vi "Add x.vi"(10 "x":sgl, 11 "Vector 2D in":refnum<class "Vector 2D.lvclass">) -> (3 "Vector 2D out":refnum<class "Vector 2D.lvclass">)   [LabVIEW 2021, in "Vector 2D.lvclass"]
uses:
  Vector 2D.lvclass
  Vector 2D.lvclass/Vector 2D.ctl
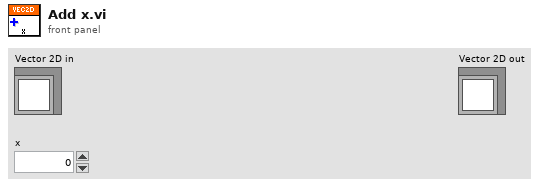
[diagram p1: front panel]
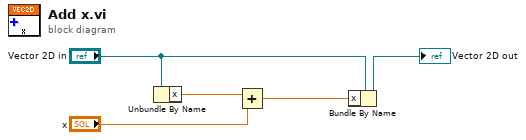
[diagram p0: block diagram]
diagram:
  n1 = Unbundle By Name("Vector 2D in") -> ("x"=w3:sgl)
  n2 = Add(x=w3, y="x") -> (x+y=w2:sgl)
  n3 = Bundle By Name(cluster="Vector 2D in", "x"=w2) -> (→"Vector 2D out":refnum<class "Vector 2D.lvclass">)
